vi "外观 1.vi"(0 "Data In":T4 caption="数据输入", 2 "Display State In":T2 caption="显示状态输入", 3 "Container State":T3 caption="容器状态") -> (6 "Data Out":T4 caption="数据输出", 7 "Display State Out":T2 caption="显示状态输出", 8 "Action":T1 caption="动作")   [LabVIEW 2016, in "多参数状态显示.xctl"]
uses:
  <vilib>/_xctls/Container State.ctl
  <vilib>/_xctls/Action.ctl
  <vilib>/_xctls/XControlSupport.lvlib
panel:
  in  "初始化 2":bool
  in  "初始化":bool
  out "数据标识":string="N"
  out "状态2":string="7.87 mg/L"
  out "状态1":string="78.56 %"
  out "标签名":string="水温"
  out "标签底板":string
  out "检测值2趋势":dbl[](array[numeric])
  out "检测值1趋势":dbl[](array[numeric])
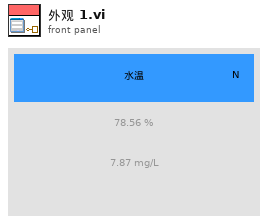
[diagram p1: front panel]
types:
  T1 = typedef "XControlSupport.lvlib/Action.ctl" = cluster{"Data Changed?":bool, "State Changed?":bool, "Action Name":string}
  T2 = typedef "多参数状态显示.xctl/状态 1.ctl" = cluster{"数值":dbl}
  T3 = typedef "XControlSupport.lvlib/Container State.ctl" = cluster{"Indicator?":bool, "Run Mode?":bool, " Refnum":refnum<vi>}
  T4 = typedef "多参数状态显示.xctl/数据 1.ctl" = cluster{"标签":string, "检测值1":cluster{"检测值":dbl, "单位":string, "启用":bool}, "检测值2":cluster{"检测值":dbl, "单位":string, "启用":bool}, "数据标识":string}
  T5 = typedef "LVPoint32TypeDef.ctl" = cluster{"Horizontal":i32, "Vertical":i32}
  T6 = typedef "LVRectTypeDef.ctl" = cluster{"Left":i16, "Top":i16, "Right":i16, "Bottom":i16}
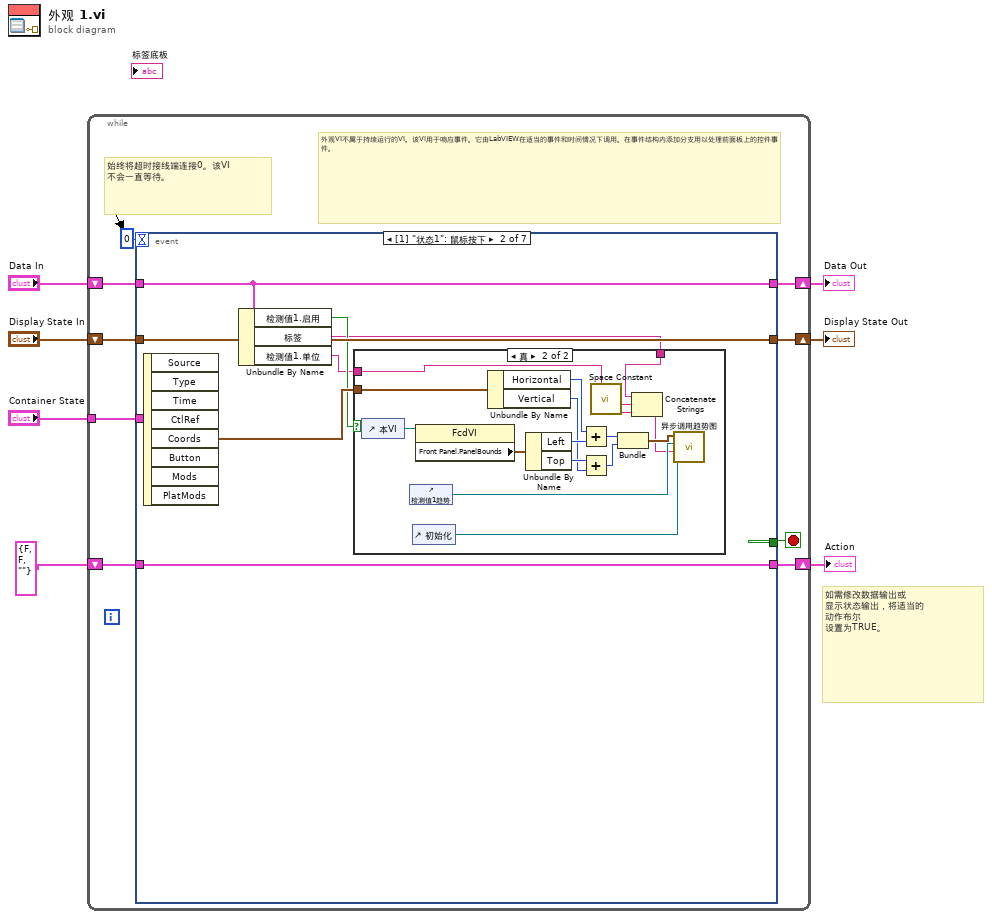
[diagram p0: block diagram]
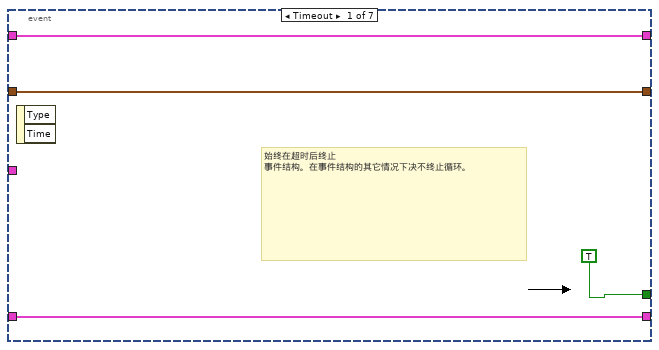
[diagram p2: hidden frame]
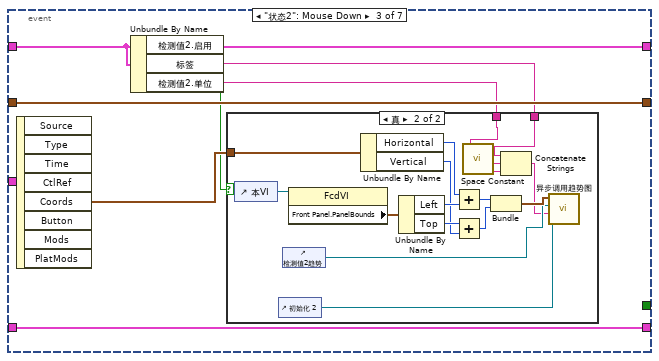
[diagram p4: hidden frame]
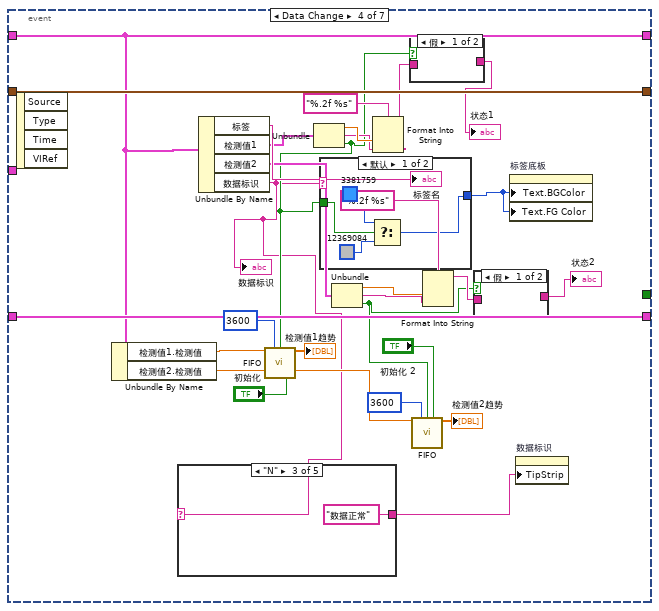
[diagram p6: hidden frame]
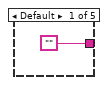
[diagram p7: hidden frame]
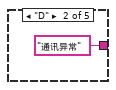
[diagram p8: hidden frame]
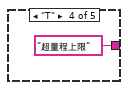
[diagram p9: hidden frame]
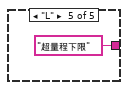
[diagram p10: hidden frame]
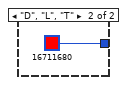
[diagram p13: hidden frame]
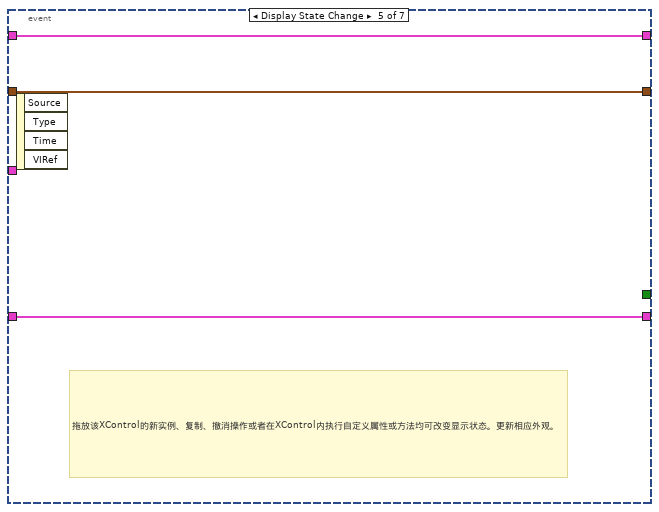
[diagram p14: hidden frame]
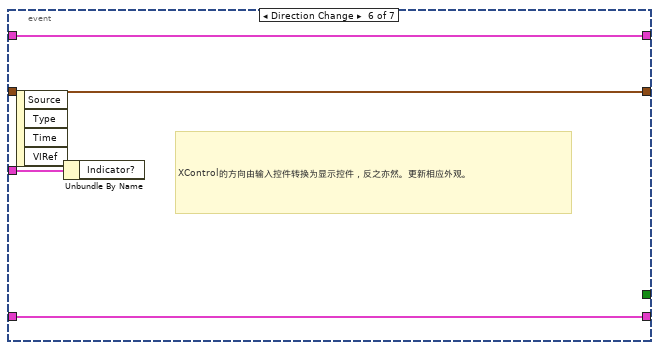
[diagram p15: hidden frame]
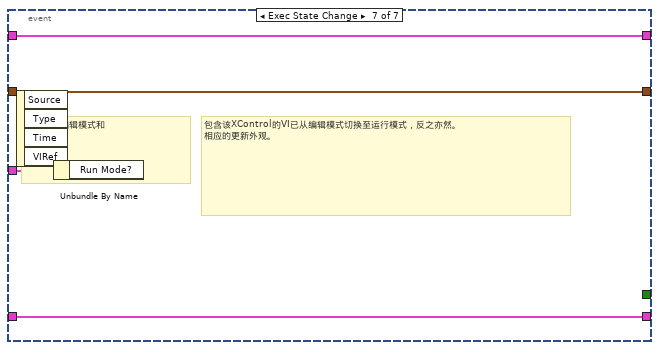
[diagram p16: hidden frame]
diagram:
  # "如需修改数据输出或\n显示状态输出，将适当的\n动作布尔\n设置为TRUE。"
  n1 = while {
    shift-right: [w15] -> w4
    shift-left: "Display State In" -> [w16]
    tunnel: "Container State" -> [w12]
    shift-right: [w10] -> w7
    shift-left: "Data In" -> [w11]
    shift-right: [w8] -> w2
    shift-left: T1 {"Data Changed?"=FALSE, "State Changed?"=FALSE, "Action Name"=""} ("Action") -> [w9]
    stop <- w14 stop-if-true
    # "外观VI不属于持续运行的VI。该VI用于响应事件。它由LabVIEW在适当的事件和时间情况下调用。在事件结构内添加分支用以处理前面板上的控件事件。"
    # "始终将超时接线端连接0。该VI\n不会一直等待。"
    n2 = event shown="[1] \"状态1\": 鼠标按下" {
      selector: _ -> [_ _ _ _ _ _ _]
      dyn-events: _ -> [_ _ _ _ _ _ _]
      timeout: 0 -> [_ _ _ _ _ _ _]
      tunnel: w16 -> [w18 w27 w50 w95 w108 w113 w117]
      tunnel: [w18 w27 w50 w95 w108 w113 w117] -> w15
      tunnel: [TRUE _ _ _ _ _ _] -> w14
      tunnel: w12 -> [_ _ _ _ _ w114 w118]
      tunnel: w11 -> [w17 w24 w47 w80 w110 w112 w116]
      tunnel: [w17 w24 w47 w80 w110 w112 w116] -> w10
      tunnel: [w19 w26 w49 w94 w109 w111 w115] -> w8
      tunnel: w9 -> [w19 w26 w49 w94 w109 w111 w115]
      event Timeout {
        # "始终在超时后终止\n事件结构。在事件结构的其它情况下决不终止循环。"
        n3 = event-data() -> ()  [unwired: 1 in, 2 out]
      }
      event "状态1": Mouse Down {
        n4 = event-data() -> ("Coords"=w25:T5)  [unwired: 1 in, 7 out]
        n5 = Unbundle By Name(w24) -> ("检测值1.启用"=w23:bool, "标签"=w22:string, "检测值1.单位"=w21:string)
        n6 = case shown="真" w23 {
          tunnel: w25 -> [_ w40]
          tunnel: w22 -> [_ w32]
          tunnel: w21 -> [_ w31]
          frame False {
          }
          frame True {
            n7 = control-ref of="本VI"() -> (w43:refnum<vi>)
            n8 = control-ref of="检测值1趋势"() -> (w33:refnum<vi>)
            n9 = control-ref of="初始化"() -> (w28:refnum<vi>)
            n10 = property class="FcdVI"(reference=w43) -> ("Front Panel.PanelBounds"=w41:T6)  [unwired: 1 in, 2 out]
            n11 = Unbundle By Name(w40) -> ("Horizontal"=w39:i32, "Vertical"=w37:i32)
            n12 = Unbundle By Name(w41) -> ("Left"=w42:i16, "Top"=w38:i16)
            n13 = Add(x=w39, y=w42) -> (x+y=w36:i32)
            n14 = Add(x=w38, y=w37) -> (x+y=w35:i32)
            n15 = call <vilib>:"Space Constant.vi"() -> ("String"=w29:string)
            n16 = Bundle(w36, w35) -> (w34:cluster{i32, i32})  [unwired: 1 in]
            n17 = Concatenate Strings(w32, w29, w31) -> (w30:string)
            n18 = call "异步调用趋势图.vi"("初始化"=w28, "参数"=w30, "Array输入"=w33, "原点"=w34) -> ()  [unwired: 8 in]
          }
        }
      }
      event "状态2": Mouse Down {
        n19 = event-data() -> ("Coords"=w48:T5)  [unwired: 1 in, 7 out]
        n20 = Unbundle By Name(w47) -> ("检测值2.启用"=w46:bool, "标签"=w45:string, "检测值2.单位"=w44:string)
        n21 = case shown="真" w46 {
          tunnel: w48 -> [_ w63]
          tunnel: w45 -> [_ w53]
          tunnel: w44 -> [_ w55]
          frame False {
          }
          frame True {
            n22 = control-ref of="本VI"() -> (w66:refnum<vi>)
            n23 = control-ref of="初始化 2"() -> (w51:refnum<vi>)
            n24 = control-ref of="检测值2趋势"() -> (w56:refnum<vi>)
            n25 = property class="FcdVI"(reference=w66) -> ("Front Panel.PanelBounds"=w64:T6)  [unwired: 1 in, 2 out]
            n26 = Unbundle By Name(w63) -> ("Horizontal"=w62:i32, "Vertical"=w60:i32)
            n27 = Unbundle By Name(w64) -> ("Left"=w65:i16, "Top"=w61:i16)
            n28 = Add(x=w62, y=w65) -> (x+y=w59:i32)
            n29 = Add(x=w61, y=w60) -> (x+y=w58:i32)
            n30 = call <vilib>:"Space Constant.vi"() -> ("String"=w52:string)
            n31 = Bundle(w59, w58) -> (w57:cluster{i32, i32})  [unwired: 1 in]
            n32 = Concatenate Strings(w53, w52, w55) -> (w54:string)
            n33 = call "异步调用趋势图.vi"("初始化"=w51, "参数"=w54, "Array输入"=w56, "原点"=w57) -> ()  [unwired: 8 in]
          }
        }
      }
      event Data Change {
        n34 = event-data() -> ()  [unwired: 1 in, 4 out]
        n35 = Unbundle By Name(w80) -> ("检测值1.检测值"=w79:dbl, "检测值2.检测值"=w77:dbl)
        n36 = Unbundle By Name(w80) -> ("标签"=→"标签名":string, "检测值1"=w92:cluster{"检测值":dbl, "单位":string, "启用":bool}, "检测值2"=w85:cluster{"检测值":dbl, "单位":string, "启用":bool}, "数据标识"=w70:string)
        "数据标识" <- w70
        n37 = case shown="\"N\"" w70 {
          tunnel: ["" "通讯异常" "数据正常" "超量程上限" "超量程下限"] -> w69
          frame Default {
          }
          frame "D" {
          }
          frame "N" {
          }
          frame "T" {
          }
          frame "L" {
          }
        }
        n38 = Unbundle(w92) -> ("检测值"=w91:dbl, "单位"=w90:string, "启用"=w72:bool)
        n39 = call "FIFO.vi"("数值"=w79, "元素大小"=u32 3600, "启用"=w72, "初始化"="初始化") -> ("数组"=→"检测值1趋势":dbl[])  [unwired: 11 in]
        n40 = case shown="默认" w70 {
          tunnel: [w103 u32 16711680] -> w71
          tunnel: w72 -> [w106 _]
          frame Default {
            n41 = Select(t=u32 3381759, s=w106, f=u32 12369084) -> (s? t:f=w103:u32)
          }
          frame "D", "L", "T" {
          }
        }
        n42 = Unbundle(w85) -> ("检测值"=w86:dbl, "单位"=w87:string, "启用"=w73:bool)
        n43 = Format Into String(format string="%.2f %s" ("格式字符串"), w91, w90) -> (resulting string=w82:string)  [unwired: 2 in, 1 out]
        n44 = case shown="假" w72 {
          tunnel: [_ w101] -> w81
          tunnel: w82 -> [_ w101]
          frame False {
          }
          frame True {
          }
        }
        "状态1" <- w81
        n45 = call "FIFO.vi"("数值"=w77, "元素大小"=u32 3600, "启用"=w73, "初始化"="初始化 2") -> ("数组"=→"检测值2趋势":dbl[])  [unwired: 11 in]
        n46 = Format Into String(format string="%.2f %s" ("格式字符串"), w86, w87) -> (resulting string=w83:string)  [unwired: 2 in, 1 out]
        n47 = case shown="假" w73 {
          tunnel: [_ w102] -> w84
          tunnel: w83 -> [_ w102]
          frame False {
          }
          frame True {
          }
        }
        "状态2" <- w84
        n48 = property on="标签底板" class="Str"("Text.BGColor"=w71, "Text.FG Color"=w71) -> ()  [unwired: 2 in, 2 out]
        n49 = property on="数据标识" class="Str"("TipStrip"=w69) -> ()  [unwired: 2 in, 2 out]
      }
      event Display State Change {
        # "拖放该XControl的新实例、复制、撤消操作或者在XControl内执行自定义属性或方法均可改变显示状态。更新相应外观。"
        n50 = event-data() -> ()  [unwired: 1 in, 4 out]
      }
      event Direction Change {
        # "XControl的方向由输入控件转换为显示控件，反之亦然。更新相应外观。"
        n51 = event-data() -> ()  [unwired: 1 in, 4 out]
        n52 = Unbundle By Name(w114) -> ()  [unwired: 1 out]
      }
      event Exec State Change {
        # "包含该XControl的VI已从编辑模式切换至运行模式，反之亦然。\n相应的更新外观。"
        # "分别处理编辑模式和\n运行模式"
        n53 = event-data() -> ()  [unwired: 1 in, 4 out]
        n54 = Unbundle By Name(w118) -> ()  [unwired: 1 out]
      }
    }
  }
  "Display State Out" <- w4
  "Data Out" <- w7
  "Action" <- w2
